vi "substring.vi"() -> ()   [LabVIEW 2017]
panel:
  out "replaced substring":string
  out "result string":string
  in  "String":string
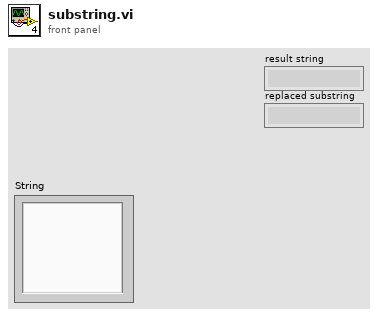
[diagram p1: front panel]
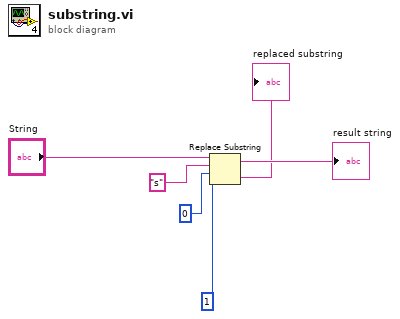
[diagram p0: block diagram]
diagram:
  n1 = Replace Substring(2:1 ("length (len. of substring)"), 3:0 ("offset (0)"), 4:"s" ("substring (\"\")"), 5:"String") -> (0:→"replaced substring":string, 1:→"result string":string)
